vi "IT6900 Step Make.vi"() -> ()   [LabVIEW 2013]
uses:
  IT6900.lvlib
panel:
  in  "Step Value":dbl=0.1 format="%.2f"
  in  "Function":u16(ring) items=["Voltage", "Current"]
  in  "Step Type":u16(ring) items=["Up", "Down"]
  in  "Serial Configuration":T1={"Baud Rate"=9600, "Parity"=0, "Data Bits"=8, "Stop Bits"=10, "Flow Control"=0} {"Flow Control" items=["None", "XON/XOFF", "RTS/CTS", "XON/XOFF & RTS/CTS", "DTR/DSR", "XON/XOFF & DTR/DSR"]; "Stop Bits" items=["1.0"=10, "1.5"=15, "2.0"=20]; "Data Bits" items=["7"=7, "8"=8]; "Parity" items=["None", "Odd", "Even", "Mark", "Space"]; "Baud Rate" items=["300"=300, "600"=600, "1200"=1200, "2400"=2400, "4800"=4800, "9600"=9600, "19200"=19200]}
  in  "Stop Output":bool
  in  "Initial Level":dbl format="%.2f"
  out "Actual Level":dbl format="%.3f"
  in  "End Level":dbl=10.0 format="%.2f"
  in  "VISA resource name":refnum<visa-resource-name>
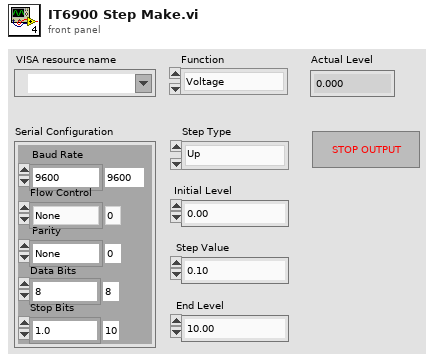
[diagram p1: front panel]
types:
  T1 = cluster{"Baud Rate":u32, "Parity":u16, "Data Bits":u16, "Stop Bits":u16, "Flow Control":u16}
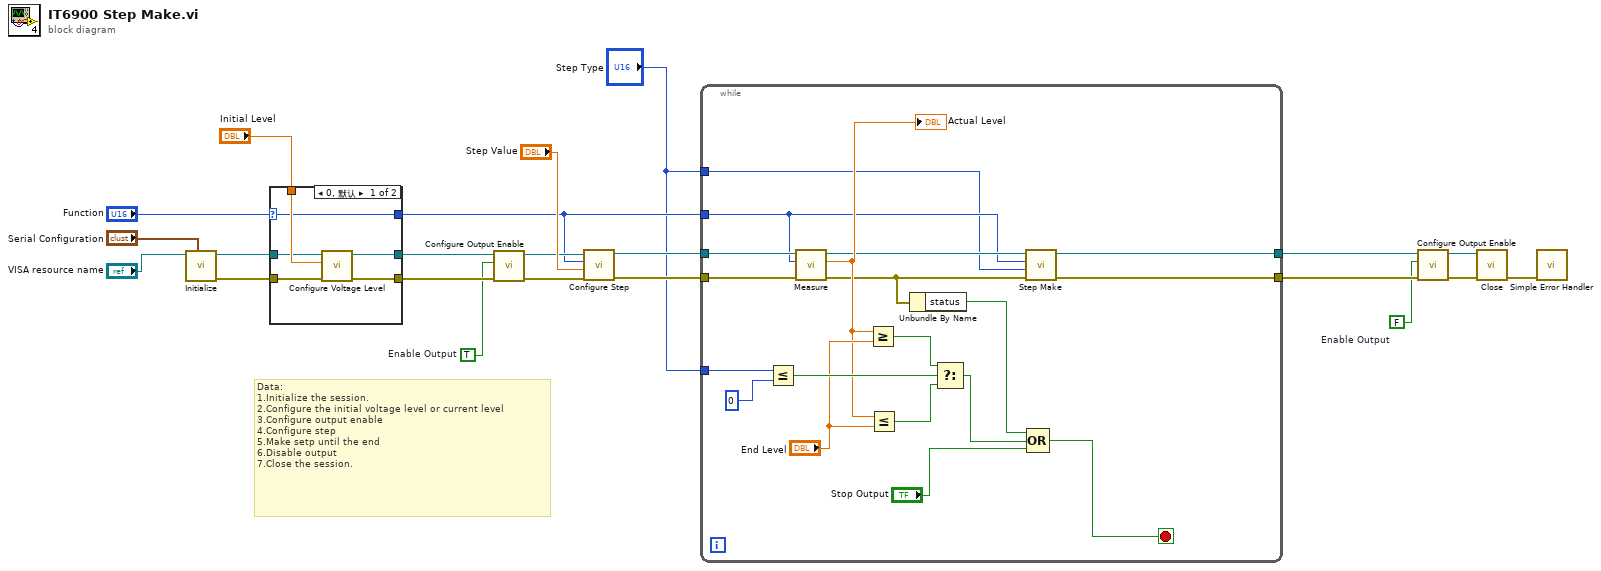
[diagram p0: block diagram]
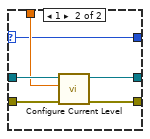
[diagram p2: hidden frame]
diagram:
  w4 = FALSE  # Enable Output
  w14 = TRUE  # Enable Output
  # "Data:\n1.Initialize the session.\n2.Configure the initial voltage level or current level\n3.Configure output enable\n4.Configure step\n5.Make setp until the end\n6.Disable output\n7.Close the session."
  n1 = call "Initialize.vi"("Serial Configuration"="Serial Configuration", "VISA resource name"="VISA resource name") -> ("error out"=w17:errorcluster, "VISA resource name out"=w18:refnum<visa-resource-name>)  [unwired: 8 in]
  n2 = case "条件结构" shown="0, 默认" "Function" {
    selector: "Function" -> [w23 w29]
    tunnel: "Initial Level" -> [w28 w32]
    tunnel: w18 -> [w27 w34]
    tunnel: w17 -> [w26 w33]
    tunnel: [w25 w31] -> w16
    tunnel: [w24 w30] -> w15
    tunnel: [w23 w29] -> w8
    frame 0, Default {
      n3 = call "Configure Voltage Level.vi"("error in (no error)"=w26, "Voltage Level (0.0 V)"=w28, "VISA resource name"=w27) -> ("error out"=w24:errorcluster, "VISA resource name out"=w25:refnum<visa-resource-name>)  [unwired: 7 in]
    }
    frame 1 {
      n4 = call "Configure Current Level.vi"("error in (no error)"=w33, "Current Level (0.0 A)"=w32, "VISA resource name"=w34) -> ("error out"=w30:errorcluster, "VISA resource name out"=w31:refnum<visa-resource-name>)  [unwired: 7 in]
    }
  }
  n5 = call "Configure Output Enable.vi"("VISA resource name"=w16, "Enable Output (T: Enable)"=w14, "error in (no error)"=w15) -> ("VISA resource name out"=w11:refnum<visa-resource-name>, "error out"=w13:errorcluster)  [unwired: 6 in]
  n6 = call "Configure Step.vi"("error in (no error)"=w13, "Step value (0.0)"="Step Value", "Function (0:Voltage)"=w8, "VISA resource name"=w11) -> ("error out"=w9:errorcluster, "VISA resource name out"=w10:refnum<visa-resource-name>)  [unwired: 6 in]
  n7 = while {
    tunnel: w10 -> [w53]
    tunnel: w9 -> [w52]
    tunnel: w8 -> [w38]
    tunnel: "Step Type" -> [w51]
    tunnel: "Step Type" -> [w37]
    tunnel: [w36] -> w6
    tunnel: [w35] -> w5
    stop <- w39 stop-if-true
    n8 = Less Or Equal?(x=w51, y=0) -> (x <= y?=w49:bool)
    n9 = call "Measure.vi"("error in (no error)"=w52, "Measure Type"=w38, "VISA resource name"=w53) -> ("error out"=w43:errorcluster, "Measurement"=w47:dbl, "VISA resource name out"=w44:refnum<visa-resource-name>)  [unwired: 6 in]
    "Actual Level" <- w47
    n10 = Greater Or Equal?(x=w47, y="End Level") -> (x >= y?=w46:bool)
    n11 = Less Or Equal?(x=w47, y="End Level") -> (x <= y?=w45:bool)
    n12 = Unbundle By Name(w43) -> ("status"=w42:bool)
    n13 = Select(t=w46, s=w49, f=w45) -> (s? t:f=w41:bool)
    n14 = call "Step Make.vi"("error in (no error)"=w43, "Step Type (0: UP)"=w37, "Function (0: Voltage)"=w38, "VISA resource name"=w44) -> ("error out"=w35:errorcluster, "VISA resource name out"=w36:refnum<visa-resource-name>)  [unwired: 6 in]
    n15 = Compound Arithmetic op=OR(w42, w41, "Stop Output") -> (w39:bool)
  }
  n16 = call "Configure Output Enable.vi"("VISA resource name"=w6, "Enable Output (T: Enable)"=w4, "error in (no error)"=w5) -> ("VISA resource name out"=w2:refnum<visa-resource-name>, "error out"=w3:errorcluster)  [unwired: 6 in]
  n17 = call "Close.vi"("error in (no error)"=w3, "VISA resource name"=w2) -> ("error out"=w1:errorcluster)  [unwired: 9 in]
  n18 = call <vilib>:"Simple Error Handler.vi"("error in (no error)"=w1) -> ()  [unwired: 4 in, 5 out]
